vi "FineReport_Update.vi"(4 "UpdataValue(array)":string[](array[string]), 5 "UpdataColumn(array)":string[](array[string]), 6 "error in (no error)":errorcluster, 7 "UpdataWhere":string, 8 "UpdataTableName":string, 9 "ADODB._Connection in":refnum<k7>) -> (0 "error out":errorcluster, 3 "ADODB._Connection Out":refnum<k7>)   [LabVIEW 2018]
panel:
  # "Rev2.0"
  # "Input"
  # "Output"
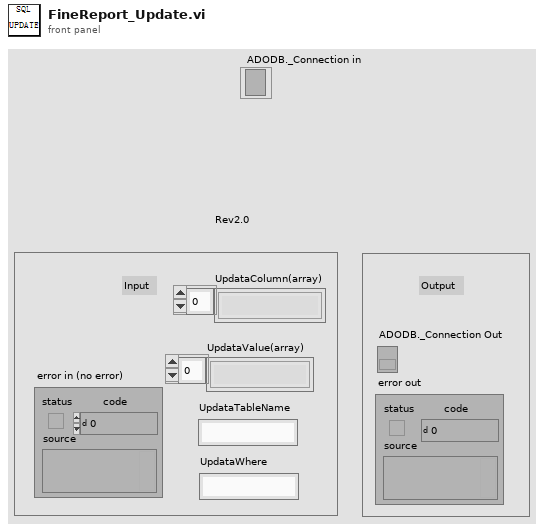
[diagram p1: front panel]
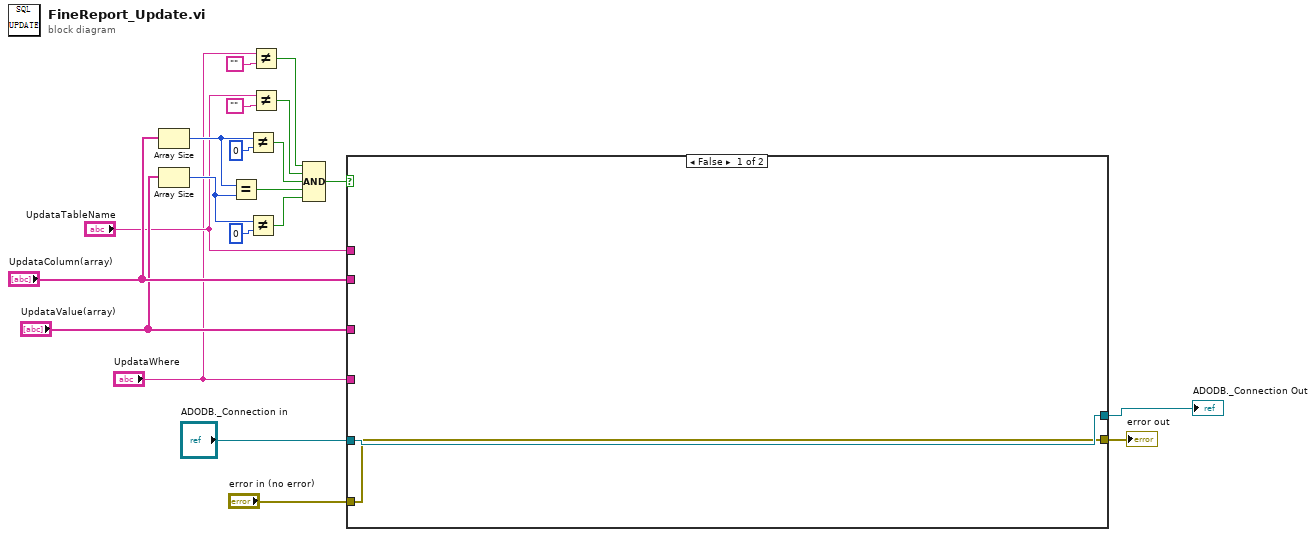
[diagram p0: block diagram]
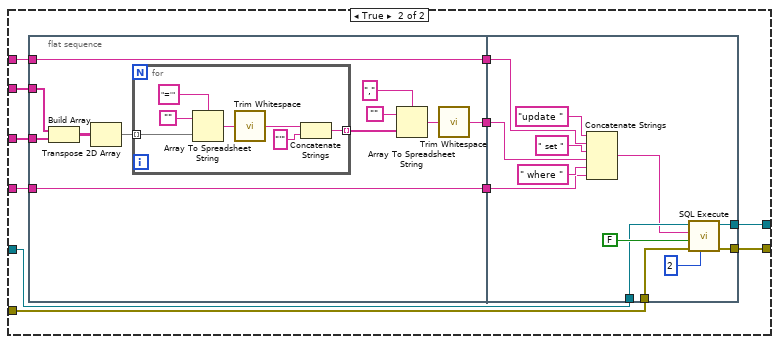
[diagram p2: hidden frame]
diagram:
  n1 = Array Size(array="UpdataColumn(array)") -> (size(s)=w14:i32)
  n2 = Array Size(array="UpdataValue(array)") -> (size(s)=w13:i32)
  n3 = Equal?(x=w14, y=w13) -> (x = y?=w9:bool)
  n4 = Not Equal?(x=w14, y=0) -> (x != y?=w10:bool)
  n5 = Not Equal?(x=w13, y=0) -> (x != y?=w8:bool)
  n6 = Not Equal?(x="UpdataWhere", y="") -> (x != y?=w12:bool)
  n7 = Not Equal?(x="UpdataTableName", y="") -> (x != y?=w11:bool)
  n8 = Compound Arithmetic op=AND(w12, w11, w10, w9, w8) -> (w7:bool)
  n9 = case shown="False" w7 {
    tunnel: "ADODB._Connection in" -> [w22 w33]
    tunnel: "error in (no error)" -> [w21 w32]
    tunnel: [w22 w31] -> w4
    tunnel: [w21 w30] -> w3
    tunnel: "UpdataColumn(array)" -> [_ w29]
    tunnel: "UpdataValue(array)" -> [_ w28]
    tunnel: "UpdataTableName" -> [_ w25]
    tunnel: "UpdataWhere" -> [_ w23]
    frame False {
    }
    frame True {
      n10 = flat-sequence {
        tunnel: w29 -> [w44]
        tunnel: w28 -> [w43]
        tunnel: [w36] -> w27
        tunnel: [w35] -> w26
        tunnel: w25 -> [w35]
        tunnel: [w34] -> w24
        tunnel: w23 -> [w34]
        tunnel: w33 -> [w62]
        tunnel: w32 -> [w61]
        tunnel: w27 -> [w57]
        tunnel: w26 -> [w56]
        tunnel: w24 -> [w55]
        tunnel: [w60] -> w31
        tunnel: [w53] -> w30
        frame #0 {
          n11 = Build Array(w44, w43) -> (w42:string[][])
          n12 = Transpose 2D Array(2D array=w42) -> (transposed array=w41:string[][])
          n13 = for {
            tunnel: w41 -> [w49] mode=indexing
            tunnel: [w47] -> w38 mode=indexing
            n14 = Array To Spreadsheet String(delimiter (Tab)="='" ("分隔符(Tab)"), array=w49, 3:"") -> (spreadsheet string=w46:string)
            n15 = call <vilib>:"Trim Whitespace.vi"("string"=w46) -> ("trimmed string"=w45:string)  [unwired: 1 in]
            n16 = Concatenate Strings(w45, "'" ("字符串")) -> (w47:string)
          }
          n17 = Array To Spreadsheet String(delimiter (Tab)="," ("分隔符(Tab)"), array=w38, 3:"") -> (spreadsheet string=w37:string)
          n18 = call <vilib>:"Trim Whitespace.vi"("string"=w37) -> ("trimmed string"=w36:string)  [unwired: 1 in]
        }
        frame #1 {
          n19 = Concatenate Strings("update ", w56, " set " ("字符串"), w57, " where " ("字符串"), w55) -> (w52:string)
          n20 = call <userlib>:"SQL Execute.vi"("Retries"=2, "error in (no error)"=w61, "Return Data (T)"=FALSE, "Command Text"=w52, "ADODB._Connection In"=w62) -> ("error out"=w53:errorcluster, "ADODB._Connection Out"=w60:refnum<k7>)  [unwired: 3 in, 2 out]
        }
      }
    }
  }
  "ADODB._Connection Out" <- w4
  "error out" <- w3
